vi "Random Competition SB.vi"() -> ()   [LabVIEW 2019]
uses:
  <vilib>/numeric/Random Number (Range) DBL.vi
panel:
  out "Winner B":bool
  out "Tie":bool
  out "Winner A":bool
  out "Points B":i32
  out "Points A":i32
  in  "Number of Iterations":i32
  out "Random Number B":dbl
  out "Random Number A":dbl
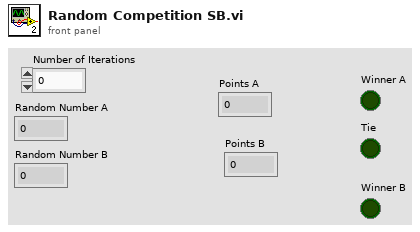
[diagram p1: front panel]
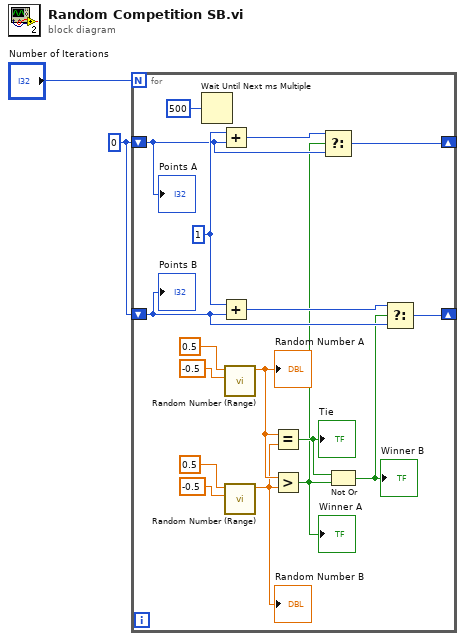
[diagram p0: block diagram]
diagram:
  w1 = 0
  n1 = for {
    N: "Number of Iterations" -> [_]
    shift-right: [w12] -> _
    shift-left: w1 -> [w7]
    shift-right: [w13] -> _
    shift-left: w1 -> [w9]
    w11 = 1
    n2 = Wait Until Next ms Multiple(millisecond multiple=u32 500) -> ()  [unwired: 1 out]
    n3 = Add(x=w11, y=w9) -> (x+y=w10:i32)
    n4 = Add(x=w11, y=w7) -> (x+y=w8:i32)
    n5 = call-poly <vilib>:"Random Number (Range).vi"("lower bound (0)"=-0.5, "upper bound (100)"=0.5) -> ("number"=w15:dbl)  [unwired: 9 in]
    "Random Number A" <- w15
    n6 = call-poly <vilib>:"Random Number (Range).vi"("lower bound (0)"=-0.5, "upper bound (100)"=0.5) -> ("number"=w14:dbl)  [unwired: 9 in]
    "Random Number B" <- w14
    n7 = Equal?(x=w15, y=w14) -> (x = y?=w5:bool)
    "Tie" <- w5
    n8 = Greater?(x=w15, y=w14) -> (0:w3:bool)
    "Winner A" <- w3
    n9 = Select(t=w10, s=w3, f=w9) -> (s? t:f=w13:i32)
    n10 = Not Or(1:w3, 2:w5) -> (0:w4:bool)
    "Winner B" <- w4
    n11 = Select(t=w8, s=w4, f=w7) -> (s? t:f=w12:i32)
    "Points A" <- w9
    "Points B" <- w7
  }
